vi "Poll Sample Transfer State.vi"(8 "error in (no error)":errorcluster, 11 "AMS Gas in":refnum<class "AMS Gas.lvclass">) -> ()   [LabVIEW 2015, in "AMS UI.lvlib" / "AMS Gas.lvclass"]
uses:
  AMS Gas.lvclass
  AMS Gas.lvclass/AMS Gas.ctl
  Controls/Sample Transfer State Enumerator.ctl
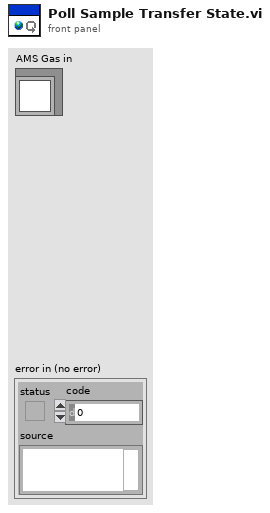
[diagram p1: front panel]
types:
  T1 = typedef "Sample Transfer State Enumerator.ctl" = enum16{"Idle", "Initialize", "Check Containers", "Check Temperatures", "Start Turbo", "Warm Up Containers", "Prepare for purging", "Purge Capillary", "Purge", "Open Containers", "Introduce Sample", "Measure Base Pressure", "Home Syringe", "Start Freezer", "Freeze Target", "Crystalize", "Initiate Stash", "Stash", "Polish", "Stop Freezers", "Push Sample", "Complete", "Abort", "Error", "Undefined"}
  T2 = typedef "FP Control Refs Cluster.ctl" = cluster{"Liquid N Valve References":T3, "Main Line Valve Refs":T4, "Transfer Line Container":refnum<vi>, "Storage Containers":refnum<vi>[], "Sample Refs":T5, "Syringe Ctrl Refs ":T6, "Baratrons Chart":refnum<vi>, "Capillary Container":refnum<vi>, "Preparation Container":refnum<vi>, "Monkey Mode":refnum<vi>}
  T3 = typedef "Liquid N Valve Ref Cluster.ctl" = cluster{"Cold Bath H2O HV 100":refnum<vi>, "Cold Bath Cleaning HV 101":refnum<vi>, "Cold Bath Storage 1 HV 102":refnum<vi>, "Cold Bath Storage 2 HV 103":refnum<vi>, "Cold Bath Storage 3 HV 104":refnum<vi>, "Cold Bath Storage 4 HV 105":refnum<vi>, "Cold Bath Syringe HV 106":refnum<vi>, "Liquid N Master Valve HV 107":refnum<vi>}
  T4 = typedef "Main Line Valve Ref Cluster.ctl" = cluster{"Turbo Valve DV313":refnum<vi>, "Prep Line Valve 0 DV300":refnum<vi>, "Storage Valves":refnum<vi>[]}
  T5 = typedef "Sample Valve Refs.ctl" = cluster{"Valves":cluster{"Sample 5 DV318":refnum<vi>, "Sample 4 DV317":refnum<vi>, "Sample 3 DV316":refnum<vi>, "Sample 2 DV315":refnum<vi>, "Sample 1 DV314":refnum<vi>}, "Lines":cluster{"Sample 1":refnum<vi>, "Sample 2":refnum<vi>, "Sample 3":refnum<vi>, "Sample 4":refnum<vi>, "Sample 5":refnum<vi>}}
  T6 = typedef "Syringe Ctrl Refs.ctl" = cluster{"Syringe Home":refnum<vi>, "Syringe Freeze":refnum<vi>, "Syringe TC":refnum<vi>, "Syringe Container":refnum<vi>}
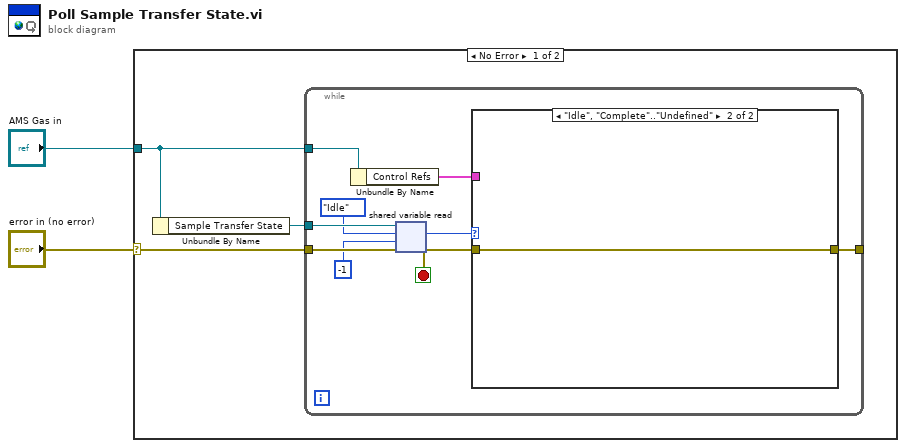
[diagram p0: block diagram]
diagram:
  n1 = case shown="No Error" "error in (no error)" {
    selector: "error in (no error)" -> [w5 _]
    tunnel: "AMS Gas in" -> [w3 _]
    frame No Error {
      n2 = Unbundle By Name(w3) -> ("Sample Transfer State"=w4:refnum<k21>)
      n3 = while {
        tunnel: w5 -> [w13]
        tunnel: w4 -> [w14]
        tunnel: w3 -> [w8]
        tunnel: [w6] -> _
        stop <- w10 stop-if-true
        n4 = Unbundle By Name(w8) -> ("Control Refs"=w7:T2)
        n5 = shared-variable-read(w14, w13, Sample_Transfer_State_Enumerator."Idle" ("Sample Transfer State"), -1 ("timeout ms")) -> (w10:errorcluster, w9:T1)  [unwired: 3 out]
        n6 = case shown="\"Idle\", \"Complete\"..\"Undefined\"" w9 {
          tunnel: w10 -> [w15 w16]
          tunnel: w7 -> [_ _]
          tunnel: [w15 w16] -> w6
          frame Default {
          }
          frame "Idle", "Complete".."Undefined" {
          }
        }
      }
    }
    frame Error {
    }
  }
